vi "iRobot Close.vi"(8 "error in":errorcluster, 11 "UART port in":T1) -> (0 "error out":errorcluster)   [LabVIEW 2015]
doc: "Stops wheels, clears UART, sets to safe mode, resets to standard baud rate, and terminates UART connection.\n\nThis VI both writes to AND reads from the serial port."
uses:
  Advanced/UART/iRobot UART Port Type.ctl
  Actuator/LED.ctl
  Advanced/Command/Baud.ctl
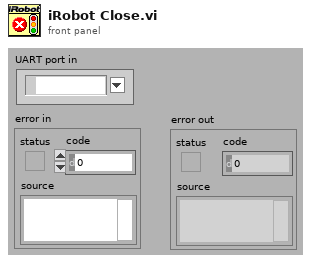
[diagram p1: front panel]
types:
  T1 = typedef "iRobot UART Port Type.ctl" = refnum<visa-resource-name>
  T2 = typedef "Baud.ctl" = enum8{"300", "600", "1200", "2400", "4800", "9600", "14400", "19200", "28800", "38400", "57600", "115200"}
  T3 = typedef "LED.ctl" = u8
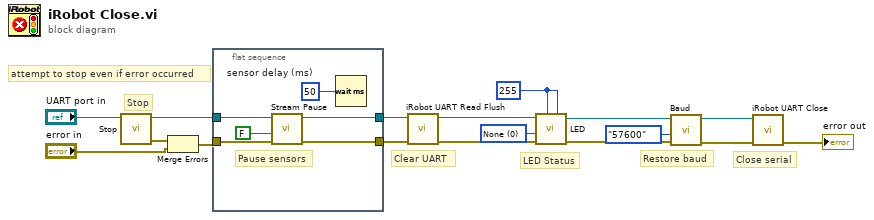
[diagram p0: block diagram]
diagram:
  w14 = T3 0 items=["None"=0, "Advance"=8, "Play"=2, "Advance + Play"=10] ("LEDs on")
  w4 = u8 255 ("Power LED Color (R-G)")
  # "attempt to stop even if error occurred"
  # "Close serial"
  # "Restore baud"
  # "Clear UART"
  # "Stop"
  # "LED Status"
  n1 = call "Stop.vi"("UART port in"="UART port in") -> ("error out"=w2:errorcluster, "UART port out"=w16:T1)  [unwired: 1 in, 8 out]
  n2 = Merge Errors(w2, "error in") -> (w1:errorcluster)
  n3 = flat-sequence {
    tunnel: w16 -> [w22]
    tunnel: [w20] -> w15
    tunnel: w1 -> [w19]
    tunnel: [w18] -> w9
    frame #0 {
      w21 = u32 50  # sensor delay (ms)
      # "Pause sensors"
      n4 = call "Stream Pause.vi"("error in"=w19, "Pause?"=FALSE ("Resume?"), "UART port in"=w22) -> ("error out"=w18:errorcluster, "UART port out"=w20:T1)  [unwired: 1 in, 6 out]
      n5 = Wait (ms)(milliseconds to wait=w21) -> ()  [unwired: 1 out]
    }
  }
  n6 = call "iRobot UART Read Flush.vi"("error in"=w9, "UART port in"=w15) -> ("error out"=w8:errorcluster, "UART port out"=w11:T1)  [unwired: 8 out]
  n7 = call "LED.vi"("Power LED Intensity (0-255)"=w4, "Power LED Color (G[0]-R[255])"=w4, "error in"=w8, "LEDs on"=w14, "UART port in"=w11) -> ("error out"=w7:errorcluster, "UART port out"=w13:T1)  [unwired: 2 in, 3 out]
  n8 = call "Baud.vi"("error in"=w7, "Baud Rate (BPS)"=Baud."57600", "UART port in"=w13) -> ("error out"=w6:errorcluster, "UART port out"=w10:T1)  [unwired: 7 out]
  n9 = call "iRobot UART Close.vi"("error in"=w6, "UART port in"=w10) -> ("error out"=→"error out":errorcluster)  [unwired: 9 out]
